vi "get piece from delivery.vi"   [LabVIEW 2018]
types:
  T1 = enum16{"shoulder", "elbow", "wrist", "base", "gripper"}
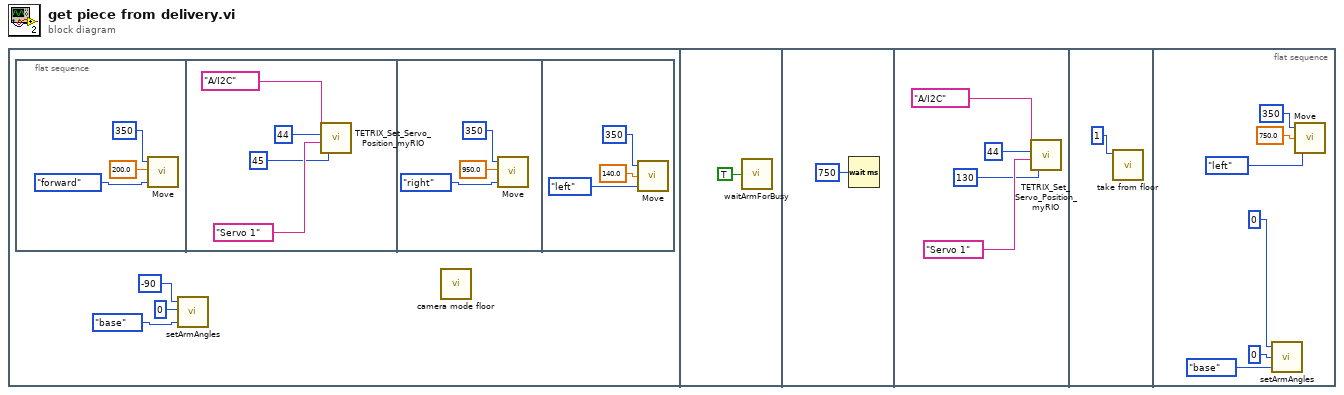
[diagram p0: block diagram]
diagram:
  n1 = flat-sequence {
    frame #0 {
      n2 = flat-sequence {
        frame #0 {
          n3 = call "Move.vi"("Enum"=enum16{"forward", "backward", "left", "right"}."forward", "distance"=200.0, "speed"=350) -> ()  [unwired: 1 in]
        }
        frame #1 {
          n4 = call <vilib>:"TETRIX_Set_Servo_Position_myRIO.vi"("myRIO MXP Port A/B"=tag "A/I2C", "Set Servo Position (0 - 180 degrees)"=u8 45, "Select Channel"="Servo 1", "Controller ID#  (I2C Address)"=u8 44) -> ()  [unwired: 3 in, 1 out]
        }
        frame #2 {
          n5 = call "Move.vi"("Enum"=enum16{"forward", "backward", "left", "right"}."right", "distance"=950.0, "speed"=350) -> ()  [unwired: 1 in]
        }
        frame #3 {
          n6 = call "Move.vi"("Enum"=enum16{"forward", "backward", "left", "right"}."left", "distance"=140.0, "speed"=350) -> ()  [unwired: 1 in]
        }
      }
      n7 = call "setArmAngles.vi"("Enum"=T1."base", "speed"=0, "angle"=-90) -> ()  [unwired: 1 in]
      n8 = call "camera mode floor.vi"() -> ()  [unwired: 12 in]
    }
    frame #1 {
      n9 = call "waitArmForBusy.vi"("base"=TRUE) -> ()
    }
    frame #2 {
      n10 = Wait (ms)(milliseconds to wait=u32 750) -> ()  [unwired: 1 out]
    }
    frame #3 {
      n11 = call <vilib>:"TETRIX_Set_Servo_Position_myRIO.vi"("myRIO MXP Port A/B"=tag "A/I2C", "Set Servo Position (0 - 180 degrees)"=u8 130, "Select Channel"="Servo 1", "Controller ID#  (I2C Address)"=u8 44) -> ()  [unwired: 3 in, 1 out]
    }
    frame #4 {
      n12 = call "take from floor.vi"("m"=1) -> ()  [unwired: 11 in]
    }
    frame #5 {
      n13 = call "setArmAngles.vi"("Enum"=T1."base", "speed"=0, "angle"=0) -> ()  [unwired: 1 in]
      n14 = call "Move.vi"("Enum"=enum16{"forward", "backward", "left", "right"}."left", "distance"=750.0, "speed"=350) -> ()  [unwired: 1 in]
    }
  }
